vi "visaRead.vi"(8 "Error in":errorcluster, 11 "VISA in":refnum<visa-resource-name>) -> (0 "Error out":errorcluster, 3 "VISA out":refnum<visa-resource-name>)   [LabVIEW 2014, in "libMux.lvlib"]
uses:
  libMux.lvlib
panel:
  out "Buffer":string
  in  "Bytes to read":u32
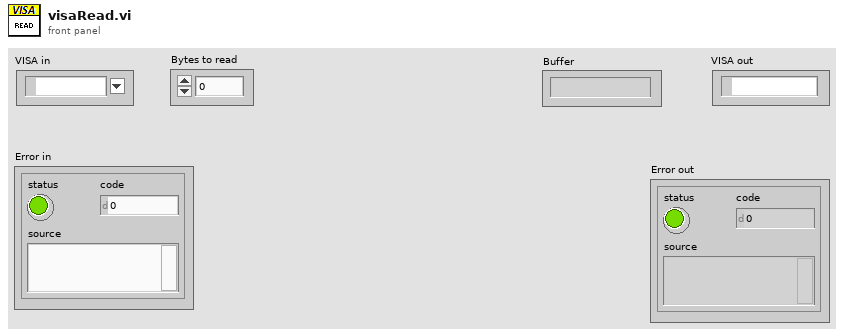
[diagram p1: front panel]
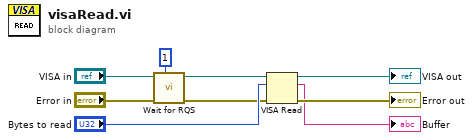
[diagram p0: block diagram]
diagram:
  n1 = call <vilib>:"Wait for RQS.vi"("timeout (25000 ms)"=u32 1, "error in (no error)"="Error in", "VISA resource name"="VISA in") -> ("error out"=w2:errorcluster, "VISA resource name out"=w8:refnum<visa-resource-name>)  [unwired: 6 in, 1 out]
  n2 = VISA Read(VISA resource name=w8, byte count="Bytes to read", error in (no error)=w2) -> (VISA resource name out=→"VISA out":refnum<visa-resource-name>, read buffer=→"Buffer":string, error out=→"Error out":errorcluster)  [unwired: 1 out]
